vi "UniqueNamesCheckAll.vi"(8 "error in (no error)":errorcluster, 11 "Devices":refnum<class "Device.lvclass">[](array[class])) -> (0 "error out":errorcluster, 3 "Devices out":refnum<class "Device.lvclass">[](array[class]))   [LabVIEW 2013]
doc: "Returns array of device names, in order of device array."
uses:
  Device/Device.lvclass
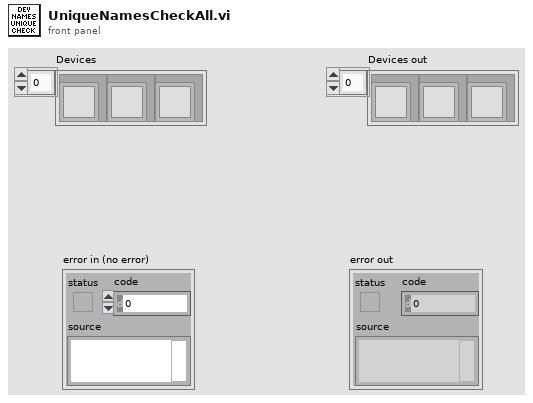
[diagram p1: front panel]
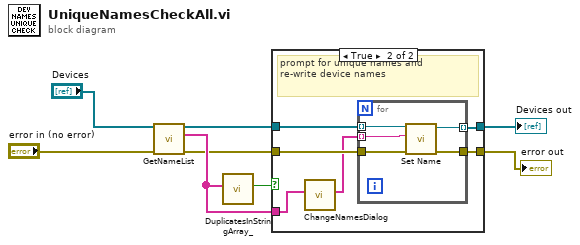
[diagram p0: block diagram]
diagram:
  n1 = call "GetNameList.vi"("error in (no error)"="error in (no error)", "Devices"="Devices") -> ("error out"=w3:errorcluster, "Names in use"=w5:string[], "Devices out"=w4:refnum<class "Device.lvclass">[])  [unwired: 7 in]
  n2 = call "DuplicatesInStringArray_.vi"("String array"=w5) -> ("duplicates?"=w6:bool)  [unwired: 10 in]
  n3 = case shown="True" w6 {
    tunnel: w5 -> [_ w16]
    tunnel: w4 -> [w10 w15]
    tunnel: w3 -> [w9 w12]
    tunnel: [w10 w14] -> w2
    tunnel: [w9 w13] -> w1
    frame False {
      # "all names are unique."
    }
    frame True {
      # "prompt for unique names and\nre-write device names"
      n4 = call "ChangeNamesDialog.vi"("Device Names"=w16) -> ("unique names"=w11:string[])  [unwired: 10 in]
      n5 = for {
        tunnel: w15 -> [w21] mode=indexing
        tunnel: [w20] -> w14 mode=indexing
        tunnel: [w19] -> w13
        tunnel: w12 -> [w18]
        tunnel: w11 -> [w17] mode=indexing
        n6 = call-dynamic "Set Name.vi"("error in (no error)"=w18, "Name"=w17, "Device in"=w21) -> ("error out"=w19:errorcluster, "Device out"=w20:refnum<class "Device.lvclass">)  [unwired: 7 in]
      }
    }
  }
  "Devices out" <- w2
  "error out" <- w1
